vi "RFmxSpecAn Meas Harms (Gmitter).vi"(1 "Reference Level (dBm)":dbl format="%.2f", 11 "error in (no error)":errorcluster) -> (15 "error out":errorcluster)   [LabVIEW 2018]
doc: "This example demonstrates the configuration of marker properties for fetching the amplitude (Y-location) and position (X-location) of a specific sample in a trace. This example also shows how to find peaks in a trace using the Marker Peak Search function."
uses:
  <instrlib>/niRFSG/niRFSG.llb/niRFSG Ref Clock Sources.ctl
  <vilib>/RFmx/SpecAn/mx/RFmxSpecAn.llb/RFmxSpecAn Select Measurement (Single).vi
  <resource>/objmgr/RFmxSpecAn.rc
  <resource>/objmgr/RFmxInstr.rc
panel:
  in  "STOP":bool
  in  "Harmonics Tab Control":enum32{"Main", "Other Config"}(tab)
  in  "SG":refnum<k15>
  in  "SG:Power (dBm)":dbl
  in  "# of Harms":i32=4 min=1 max=10
  in  "SA":refnum<k15> caption="Resource Name"
  in  "Frequency Source":string(combo)="OnboardClock"
  in  "Frequency (Hz)":dbl=10000000.0 format="%.6p"
  in  "AveragingType":i32(ring) items=["RMS", "Log", "Scalar", "Max", "Min", "Vector"]
  in  "Averaging Enabled":i32(ring) items=["False", "True"]
  in  "Averaging Count":i32=10
  in  "ref clock source":T1="OnboardClock"
  in  "ref clock rate (Hz)":dbl(ring)=10000000.0 items=["Auto"=-1.0, "10MHz"=10000000.0]
  out "Marker Level":dbl format="%.2f"
  out "Marker Freq":dbl format="%#_6p"
  out "Spectrum":cluster{"x0":dbl, "dx":dbl, "y":sgl[]}(graph)={"x0"=999500000.0, "dx"=1000.0, "y"=[]}
  # "Frequency Reference"
  # "Averaging"
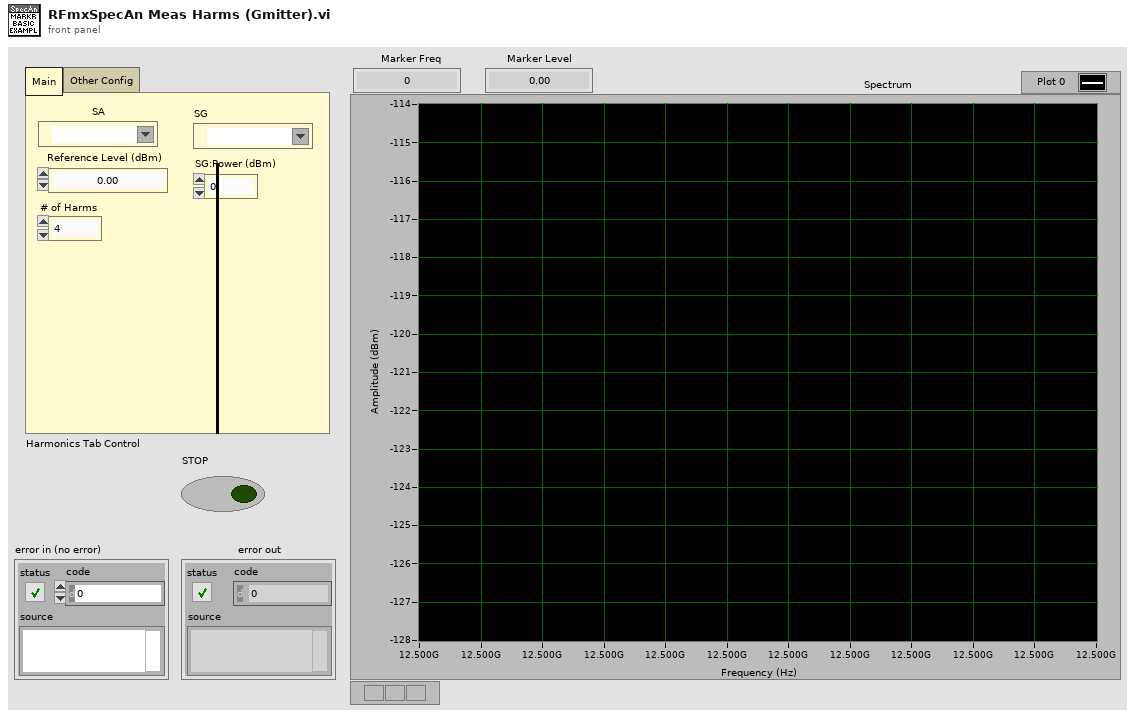
[diagram p1: front panel]
types:
  T1 = typedef "niRFSG Ref Clock Sources.ctl" = string
  T2 = enum16{"ACP", "CCDF", "CHP", "FCnt", "Harmonics", "OBW", "SEM", "Spectrum", "Spur", "TXP", "AMPM", "DPD", "IQ", "IM", "NF", "PhaseNoise"}
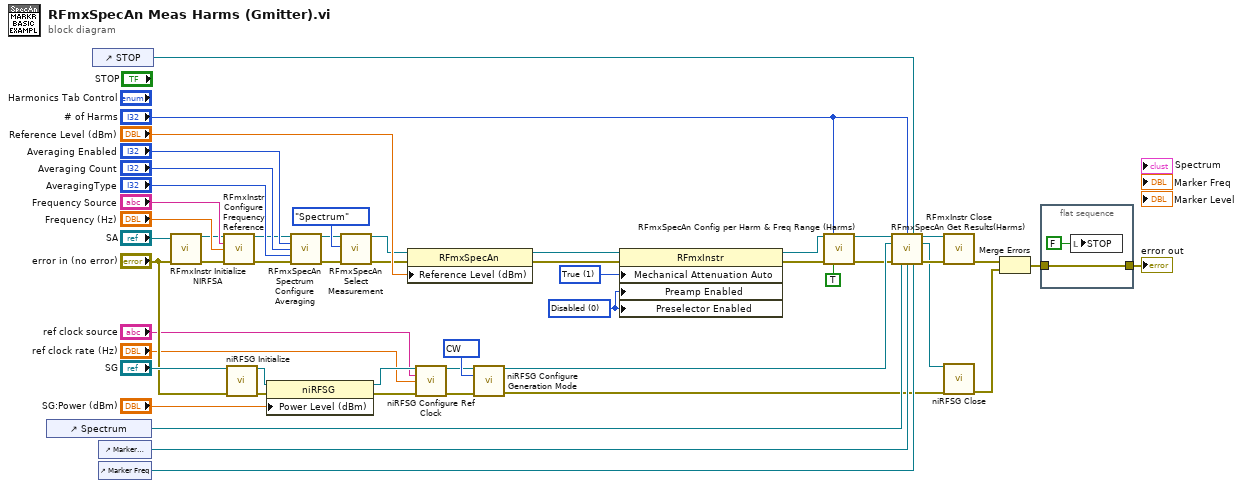
[diagram p0: block diagram]
diagram:
  w15 = 0 items=["Disabled"=0, "Enabled"=1, "Automatic"=3] ("Preamp Enabled")
  w7 = 1 items=["False", "True"] ("Mechanical Attenuation Auto")
  w38 = 1000 items=["CW"=1000, "Arb Waveform"=1001, "Script"=1002] ("generation mode")
  n1 = control-ref of="Spectrum"() -> (w35:refnum<vi>)
  n2 = control-ref of="STOP"() -> (w6:refnum<vi>)
  n3 = control-ref of="Marker Level"() -> (w34:refnum<vi>)
  n4 = control-ref of="Marker Freq"() -> (w33:refnum<vi>)
  n5 = call <vilib>:"RFmxInstr Initialize NIRFSA.vi"("Resource Name"="SA", "error in (no error)"="error in (no error)") -> ("Instrument Handle Out"=w23:refnum<k21>, "error out"=w22:errorcluster)  [unwired: 11 in, 1 out]
  n6 = call <vilib>:"RFmxInstr Configure Frequency Reference.vi"("Instrument Handle In"=w23, "Frequency Reference Source"="Frequency Source", "Frequency (Hz)"="Frequency (Hz)", "error in (no error)"=w22) -> ("Instrument Handle Out"=w45:refnum<k21>, "error out"=w44:errorcluster)  [unwired: 10 in]
  n7 = call <instrlib>:"niRFSG Initialize.vi"("resource name"="SG", "error in"="error in (no error)") -> ("instrument handle"=w29:refnum<k15>, "error out"=w40:errorcluster)  [unwired: 12 in]
  n8 = property class="niRFSG"(reference=w29, error in=w40, "Power Level (dBm)"="SG:Power (dBm)") -> (reference out=w11:refnum<k15>, error out=w12:errorcluster)
  n9 = call <vilib>:"RFmxSpecAn Spectrum Configure Averaging.vi"("Instrument Handle In"=w45, "Averaging Enabled"="Averaging Enabled", "Averaging Count"="Averaging Count", "Averaging Type"="AveragingType", "error in (no error)"=w44) -> ("Instrument Handle Out"=w43:refnum<k21>, "error out"=w42:errorcluster)  [unwired: 9 in]
  n10 = call-poly <vilib>:"RFmxSpecAn Select Measurement.vi"("Instrument Handle In"=w43, "Measurement"=T2."Spectrum", "error in (no error)"=w42) -> ("Instrument Handle Out"=w2:refnum<k21>, "error out"=w10:errorcluster)  [unwired: 11 in]
  n11 = property class="RFmxSpecAn"(reference=w2, error in=w10, "Reference Level (dBm)"="Reference Level (dBm)") -> (reference out=w25:refnum<k21>, error out=w26:errorcluster)
  n12 = call <instrlib>:"niRFSG Configure Ref Clock.vi"("instrument handle"=w11, "ref clock source"="ref clock source", "ref clock rate (Hz)"="ref clock rate (Hz)", "error in"=w12) -> ("instrument handle out"=w14:refnum<k15>, "error out"=w13:errorcluster)  [unwired: 10 in]
  n13 = call <instrlib>:"niRFSG Configure Generation Mode.vi"("instrument handle"=w14, "generation mode"=w38, "error in"=w13) -> ("instrument handle out"=w27:refnum<k15>, "error out"=w31:errorcluster)  [unwired: 11 in]
  n14 = property class="RFmxInstr"(reference=w25, error in=w26, "Mechanical Attenuation Auto"=w7, "Preamp Enabled"=w15, "Preselector Enabled"=w15) -> (reference out=w19:refnum<k21>, error out=w21:errorcluster)
  n15 = call "RFmxSpecAn Config per Harm & Freq Range (Harms).vi"("SA Handle In"=w19, "# of Harms"="# of Harms", "error in (no error)"=w21, "Read Config File"=TRUE) -> ("SA Handle Out"=w18:refnum<k21>, "error out"=w20:errorcluster)  [unwired: 9 in, 1 out]
  n16 = call "RFmxSpecAn Get Results(Harms).vi"("SA Handle In"=w18, "# of Harms"="# of Harms", "STOP"=w6, "SG Handle In"=w27, "error in (no error)"=w20, "Spectrum"=w35, "Marker Level"=w34, "Marker Freq"=w33) -> ("SA Handle Out"=w1:refnum<k21>, "SG handle out"=w30:refnum<k15>, "error out"=w36:errorcluster)  [unwired: 5 in]
  n17 = call <vilib>:"RFmxInstr Close.vi"("Instrument Handle In"=w1, "error in (no error)"=w36) -> ("error out"=w37:errorcluster)  [unwired: 13 in]
  n18 = call <instrlib>:"niRFSG Close.vi"("instrument handle"=w30, "error in"=w31) -> ("error out"=w32:errorcluster)  [unwired: 13 in]
  n19 = Merge Errors(w37, w32) -> (w5:errorcluster)
  n20 = flat-sequence {
    tunnel: w5 -> [w53]
    tunnel: [w53] -> w4
    frame #0 {
      n21 = local write "STOP"(FALSE ("STOP")) -> ()
    }
  }
  "error out" <- w4
